vi "Set next state.vi"(6 "Last Carrier?":bool, 7 "Last Measurement":bool, 9 "Last Frequency?":bool, 10 "Last Power?":bool, 11 "Last setting":bool) -> (3 "Run States":T1)   [LabVIEW 2020, in "MCCW ACLR.lvclass"]
uses:
  MCCW ACLR.lvclass
  Controls/Run States.ctl
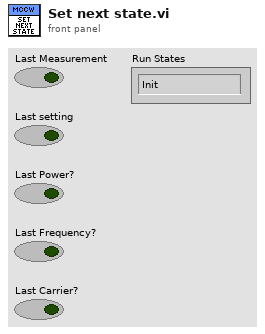
[diagram p1: front panel]
types:
  T1 = typedef "MCCW ACLR.lvclass/Run States.ctl" = enum16{"Init", "Set Frequency", "Set Power", "Set Carriers", "Set Device", "Set Measurement Number", "Measure", "Done"}
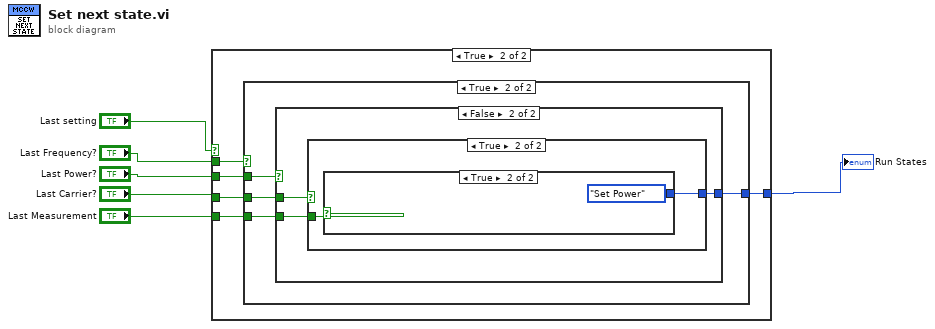
[diagram p0: block diagram]
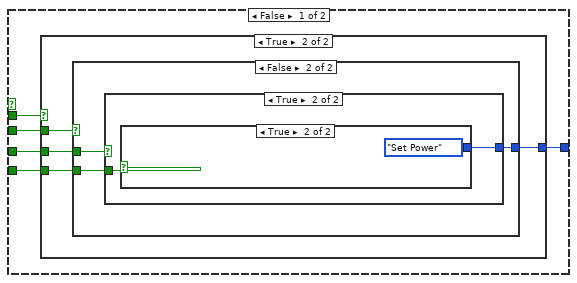
[diagram p2: hidden frame]
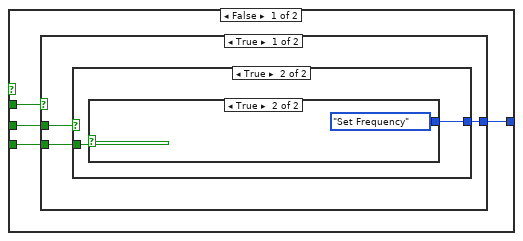
[diagram p3: hidden frame]
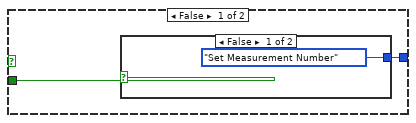
[diagram p4: hidden frame]
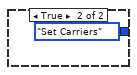
[diagram p5: hidden frame]
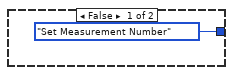
[diagram p6: hidden frame]
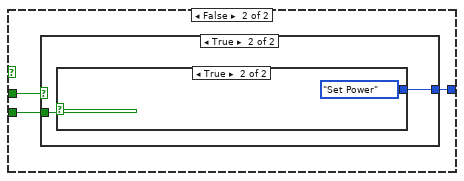
[diagram p7: hidden frame]
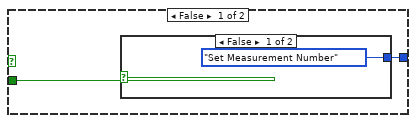
[diagram p8: hidden frame]
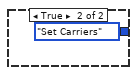
[diagram p9: hidden frame]
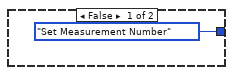
[diagram p10: hidden frame]
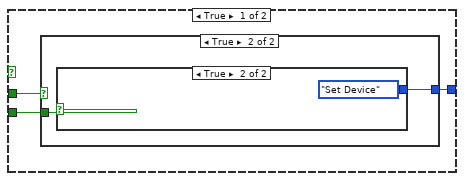
[diagram p11: hidden frame]
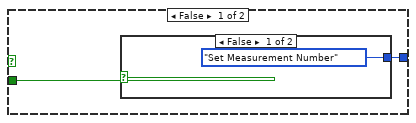
[diagram p12: hidden frame]
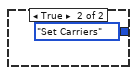
[diagram p13: hidden frame]
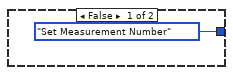
[diagram p14: hidden frame]
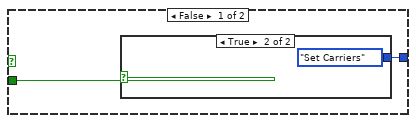
[diagram p15: hidden frame]
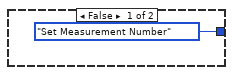
[diagram p16: hidden frame]
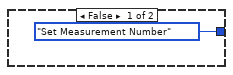
[diagram p17: hidden frame]
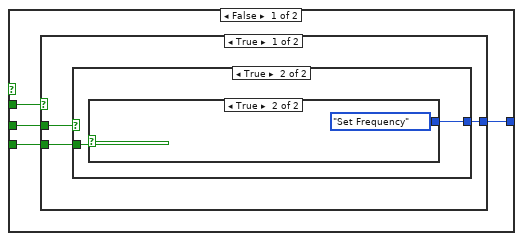
[diagram p18: hidden frame]
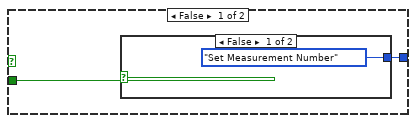
[diagram p19: hidden frame]
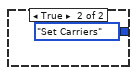
[diagram p20: hidden frame]
diagram:
  n1 = case shown="True" "Last setting" {
    tunnel: "Last Frequency?" -> [w11 w68]
    tunnel: "Last Power?" -> [w10 w67]
    tunnel: [w9 w66] -> w2
    tunnel: "Last Carrier?" -> [w8 w65]
    tunnel: "Last Measurement" -> [w7 w64]
    frame False {
      n2 = case shown="True" w11 {
        tunnel: w10 -> [w15 w41]
        tunnel: [w14 w40] -> w9
        tunnel: w8 -> [w13 w39]
        tunnel: w7 -> [w12 w38]
        frame False {
          n3 = case shown="True" w15 {
            tunnel: [w18 w29] -> w14
            tunnel: w13 -> [w17 w28]
            tunnel: w12 -> [w16 w27]
            frame True {
              n4 = case shown="True" w17 {
                tunnel: [w20 w23] -> w18
                tunnel: w16 -> [w19 w24]
                frame False {
                  n5 = case shown="False" w19 {
                    tunnel: [Run_States."Set Measurement Number" ("Run States") Run_States."Set Carriers" ("Run States")] -> w20
                    frame False {
                    }
                    frame True {
                    }
                  }
                }
                frame True {
                  n6 = case shown="True" w24 {
                    tunnel: [Run_States."Set Measurement Number" ("Run States") Run_States."Set Frequency" ("Run States")] -> w23
                    frame False {
                    }
                    frame True {
                    }
                  }
                }
              }
            }
            frame False {
              n7 = case shown="True" w28 {
                tunnel: [w31 w34] -> w29
                tunnel: w27 -> [w30 w35]
                frame False {
                  n8 = case shown="False" w30 {
                    tunnel: [Run_States."Set Measurement Number" ("Run States") Run_States."Set Carriers" ("Run States")] -> w31
                    frame False {
                    }
                    frame True {
                    }
                  }
                }
                frame True {
                  n9 = case shown="True" w35 {
                    tunnel: [Run_States."Set Measurement Number" ("Run States") Run_States."Set Power" ("Run States")] -> w34
                    frame False {
                    }
                    frame True {
                    }
                  }
                }
              }
            }
          }
        }
        frame True {
          n10 = case shown="False" w41 {
            tunnel: [w44 w55] -> w40
            tunnel: w39 -> [w43 w54]
            tunnel: w38 -> [w42 w53]
            frame True {
              n11 = case shown="True" w43 {
                tunnel: [w46 w49] -> w44
                tunnel: w42 -> [w45 w50]
                frame False {
                  n12 = case shown="False" w45 {
                    tunnel: [Run_States."Set Measurement Number" ("Run States") Run_States."Set Carriers" ("Run States")] -> w46
                    frame False {
                    }
                    frame True {
                    }
                  }
                }
                frame True {
                  n13 = case shown="True" w50 {
                    tunnel: [Run_States."Set Measurement Number" ("Run States") Run_States."Set Device" ("Run States")] -> w49
                    frame False {
                    }
                    frame True {
                    }
                  }
                }
              }
            }
            frame False {
              n14 = case shown="True" w54 {
                tunnel: [w57 w60] -> w55
                tunnel: w53 -> [w56 w61]
                frame False {
                  n15 = case shown="True" w56 {
                    tunnel: [Run_States."Set Measurement Number" ("Run States") Run_States."Set Carriers" ("Run States")] -> w57
                    frame False {
                    }
                    frame True {
                    }
                  }
                }
                frame True {
                  n16 = case shown="True" w61 {
                    tunnel: [Run_States."Set Measurement Number" ("Run States") Run_States."Set Power" ("Run States")] -> w60
                    frame False {
                    }
                    frame True {
                    }
                  }
                }
              }
            }
          }
        }
      }
    }
    frame True {
      n17 = case shown="True" w68 {
        tunnel: w67 -> [w72 w98]
        tunnel: [w71 w97] -> w66
        tunnel: w65 -> [w70 w96]
        tunnel: w64 -> [w69 w95]
        frame False {
          n18 = case shown="True" w72 {
            tunnel: [w75 w86] -> w71
            tunnel: w70 -> [w74 w85]
            tunnel: w69 -> [w73 w84]
            frame True {
              n19 = case shown="True" w74 {
                tunnel: [w77 w80] -> w75
                tunnel: w73 -> [w76 w81]
                frame False {
                  n20 = case shown="False" w76 {
                    tunnel: [Run_States."Set Measurement Number" ("Run States") Run_States."Set Carriers" ("Run States")] -> w77
                    frame False {
                    }
                    frame True {
                    }
                  }
                }
                frame True {
                  n21 = case shown="True" w81 {
                    tunnel: [Run_States."Set Measurement Number" ("Run States") Run_States."Set Frequency" ("Run States")] -> w80
                    frame False {
                    }
                    frame True {
                    }
                  }
                }
              }
            }
            frame False {
              n22 = case shown="True" w85 {
                tunnel: [w88 w91] -> w86
                tunnel: w84 -> [w87 w92]
                frame False {
                  n23 = case shown="False" w87 {
                    tunnel: [Run_States."Set Measurement Number" ("Run States") Run_States."Set Carriers" ("Run States")] -> w88
                    frame False {
                    }
                    frame True {
                    }
                  }
                }
                frame True {
                  n24 = case shown="True" w92 {
                    tunnel: [Run_States."Set Measurement Number" ("Run States") Run_States."Set Power" ("Run States")] -> w91
                    frame False {
                    }
                    frame True {
                    }
                  }
                }
              }
            }
          }
        }
        frame True {
          n25 = case shown="False" w98 {
            tunnel: [w101 w112] -> w97
            tunnel: w96 -> [w100 w111]
            tunnel: w95 -> [w99 w110]
            frame True {
              n26 = case shown="True" w100 {
                tunnel: [w103 w106] -> w101
                tunnel: w99 -> [w102 w107]
                frame False {
                  n27 = case shown="False" w102 {
                    tunnel: [Run_States."Set Measurement Number" ("Run States") Run_States."Set Carriers" ("Run States")] -> w103
                    frame False {
                    }
                    frame True {
                    }
                  }
                }
                frame True {
                  n28 = case shown="True" w107 {
                    tunnel: [Run_States."Set Measurement Number" ("Run States") Run_States."Done" ("Run States")] -> w106
                    frame False {
                    }
                    frame True {
                    }
                  }
                }
              }
            }
            frame False {
              n29 = case shown="True" w111 {
                tunnel: [w114 w117] -> w112
                tunnel: w110 -> [w113 w118]
                frame False {
                  n30 = case shown="True" w113 {
                    tunnel: [Run_States."Set Measurement Number" ("Run States") Run_States."Set Carriers" ("Run States")] -> w114
                    frame False {
                    }
                    frame True {
                    }
                  }
                }
                frame True {
                  n31 = case shown="True" w118 {
                    tunnel: [Run_States."Set Measurement Number" ("Run States") Run_States."Set Power" ("Run States")] -> w117
                    frame False {
                    }
                    frame True {
                    }
                  }
                }
              }
            }
          }
        }
      }
    }
  }
  "Run States" <- w2
